vi "Demo1 (FPGA).vi"   [LabVIEW 2012]
uses:
  <vilib>/rvi/Emulation/niFpgaSctlEmulationGetInTimedLoop.vi
  <vilib>/rvi/DataTransferAndStorage/Container/Common/niFpgaContainerGetUniqueNameForEmu.vi
  <vilib>/rvi/FIFO/Fifo_Resource/nirvififoEmulationSetSize.vi
  <vilib>/rvi/Emulation/niFpgaSctlEmulationFifoFullMgr.vi
  <vilib>/rvi/errors/niFpgaSetErrorForExecOnDevCompSimple.vi
  <vilib>/rvi/eio/common/nirviEmuReportErrorAndStop.vi
  <vilib>/rvi/interface/RandomDataEmulation/nirviRandomDataFPGAFIFO.vi
  <vilib>/rvi/interface/RandomDataEmulation/niFpgaRandomDataHandleErrors.vi
  Instance           1 20Saved   Demo1 (FPGA) .vi
  <vilib>/rvi/eio/common/nirviEmuTemplateMethod_errors.vi
  <vilib>/rvi/Emulation/niFpgaSctlEmulationResourceMgr.vi
  <vilib>/rvi/DataTransferAndStorage/Container/XNode/niFpgaContainer.xnode
  <vilib>/rvi/FIFO/Fifo_Resource/nirvififoEmulationRead.vi
  <vilib>/rvi/interface/RandomDataEmulation/nirviRandomDataFpgaReadWriteTemplate.vi
  <vilib>/eio/EIONode/EIONode.xnode
  <vilib>/rvi/FIFO/Fifo_Resource/nirvififoEmulationWrite.vi
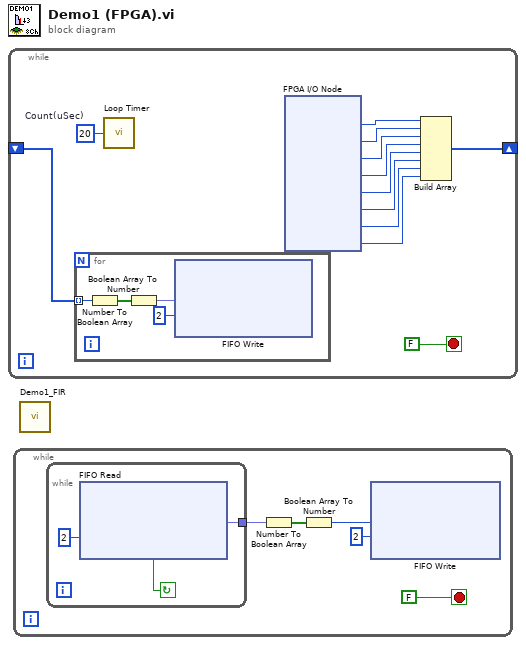
[diagram p0: block diagram]
diagram:
  n1 = while {
    shift-right: [w3] -> _
    shift-left: _ -> [w2]
    stop <- FALSE stop-if-true
    w1 = u16 20  # Count(uSec)
    n2 = for {
      tunnel: w2 -> [w15] mode=indexing
      n3 = Number To Boolean Array(number=w15) -> (Boolean array=w14:bool[])
      n4 = Boolean Array To Number(Boolean array=w14) -> (number=w13:fxp<+/-,16,1>)
      n5 = xnode ("FIFO Write")("Element"=w13, "Timeout"=2) -> ()  [unwired: 1 in, 2 out]
    }
    n6 = call "Loop Timer"("Count(uSec)"=w1) -> ()  [unwired: 1 out]
    n7 = xnode "FPGA I/O Node"() -> ("AI0"=w11:i16, "AI1"=w10:i16, "AI2"=w9:i16, "AI3"=w8:i16, "AI4"=w7:i16, "AI5"=w6:i16, "AI6"=w5:i16, "AI7"=w4:i16)  [unwired: 8 in, 8 out]
    n8 = Build Array(w11, w10, w9, w8, w7, w6, w5, w4) -> (w3:i16[])
  }
  n9 = while {
    stop <- FALSE stop-if-true
    n10 = while {
      tunnel: [w23] -> w19
      stop <- w22 continue-if-true
      n11 = xnode ("FIFO Read")("Timeout"=2) -> ("Element"=w23:fxp<+/-,16,2>, "Timed Out?"=w22:bool)  [unwired: 1 in, 1 out]
    }
    n12 = Number To Boolean Array(number=w19) -> (Boolean array=w18:bool[])
    n13 = Boolean Array To Number(Boolean array=w18) -> (number=w17:i16)
    n14 = xnode ("FIFO Write")("Element"=w17, "Timeout"=2) -> ()  [unwired: 1 in, 2 out]
  }
  n15 = call "Demo1_FIR.vi"() -> ()  [unwired: 1 out]
